vi "BalancePressure4a.vi"(0 "FirgelliError":errorcluster, 1 "length":dbl=50.0 caption="Actuator Length (mm)", 2 "DesiredPressure":dbl=-0.08 min=-1.0 max=0.0 step=0.001, 3 "Position (mm)":dbl(slide)=25.0 min=0.0 max=50.0 step=0.2 scale=0.0..50.0 scale format="%.2f", 4 "ArduinoHandle":T2={"VISA resource"="", "Board Type"=enum."Uno", "Connection Type"=enum."USB / Serial", "Bytes Per Packet (15)"=15}, 5 "CurrentPressure":dbl, 6 "WRITE_HANDLE":u32 format="%04x", 7 "PressureOffset":dbl, 8 "READ_HANDLE":u32 format="%04x", 9 "Control Values":T1, 10 "Transducer (psi)":dbl(ring)=1.0 items=["+/- .18 psi"=1.0, "+/- .36 psi"=2.0, "+/- 1.08 psi"=3.0], 11 "Syringe (mL)":dbl(ring)=1.0 items=[".5 mL"=2.0, "1 mL"=1.0, "3 mL"=3.0]) -> (14 "FirgelliError Out":errorcluster, 15 "Control Values Out":T1, 16 "UpdateChart?":bool, 17 "Position (mm) Out":dbl(slide)=25.0 min=0.0 max=50.0 step=0.2 scale=0.0..50.0 scale format="%.2f", 18 "ArduinoError Out":errorcluster, 19 "Pressure (psi)":dbl)   [LabVIEW 2011]
uses:
  <vilib>/LabVIEW Interface for Arduino/Type Defs/Arduino Resource.ctl
  <vilib>/LabVIEW Interface for Arduino/Type Defs/Board Type.ctl
  orders/Firgelli motor/LAC_Software_V2/Firgelli Labview Example/Firgelli_LAC_LabVIEWsourceVer8_2/typeDefs/controlValues.ctl
  <vilib>/LabVIEW Interface for Arduino/LabVIEW Interface for Arduino.lvlib
panel:
  in  "Accuracy":dbl
  in  "P":dbl=4.0
  in  "stop 2":bool
  in  "stop":bool
  in  "D":dbl
  in  "I":dbl
  out "LastError":dbl
  out "Error":dbl
  out "LastPressure":dbl
  in  "ArduinoError":errorcluster
  in  "Analog Input Pin (0)":u8=1
  in  "Valve I/O Pin":u8=2
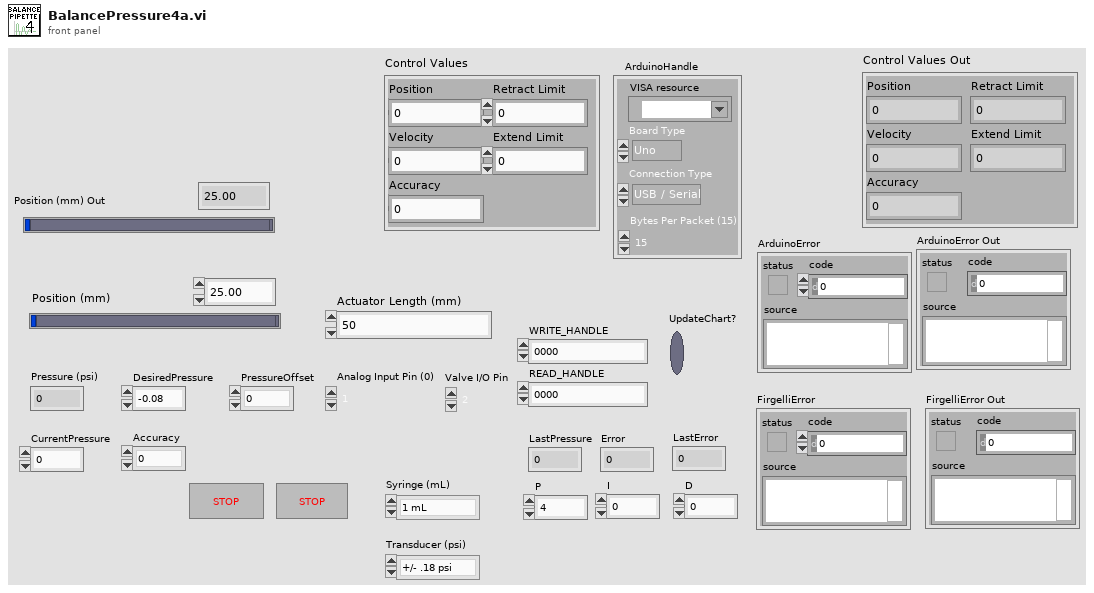
[diagram p1: front panel]
types:
  T1 = typedef "controlValues.ctl" = cluster{"Position":u16, "Velocity":u16, "Accuracy":u16, "Retract Limit":u16, "Extend Limit":u16}
  T2 = typedef "LabVIEW Interface for Arduino.lvlib/Arduino Resource.ctl" = cluster{"VISA resource":refnum<visa-resource-name>, "Board Type":T3, "Connection Type":enum8{"USB / Serial"}, "Bytes Per Packet (15)":u8}
  T3 = typedef "LabVIEW Interface for Arduino.lvlib/Board Type.ctl" = enum16{"Uno", "Dimuelanove w/Atmega 328", "Mega 2560"}
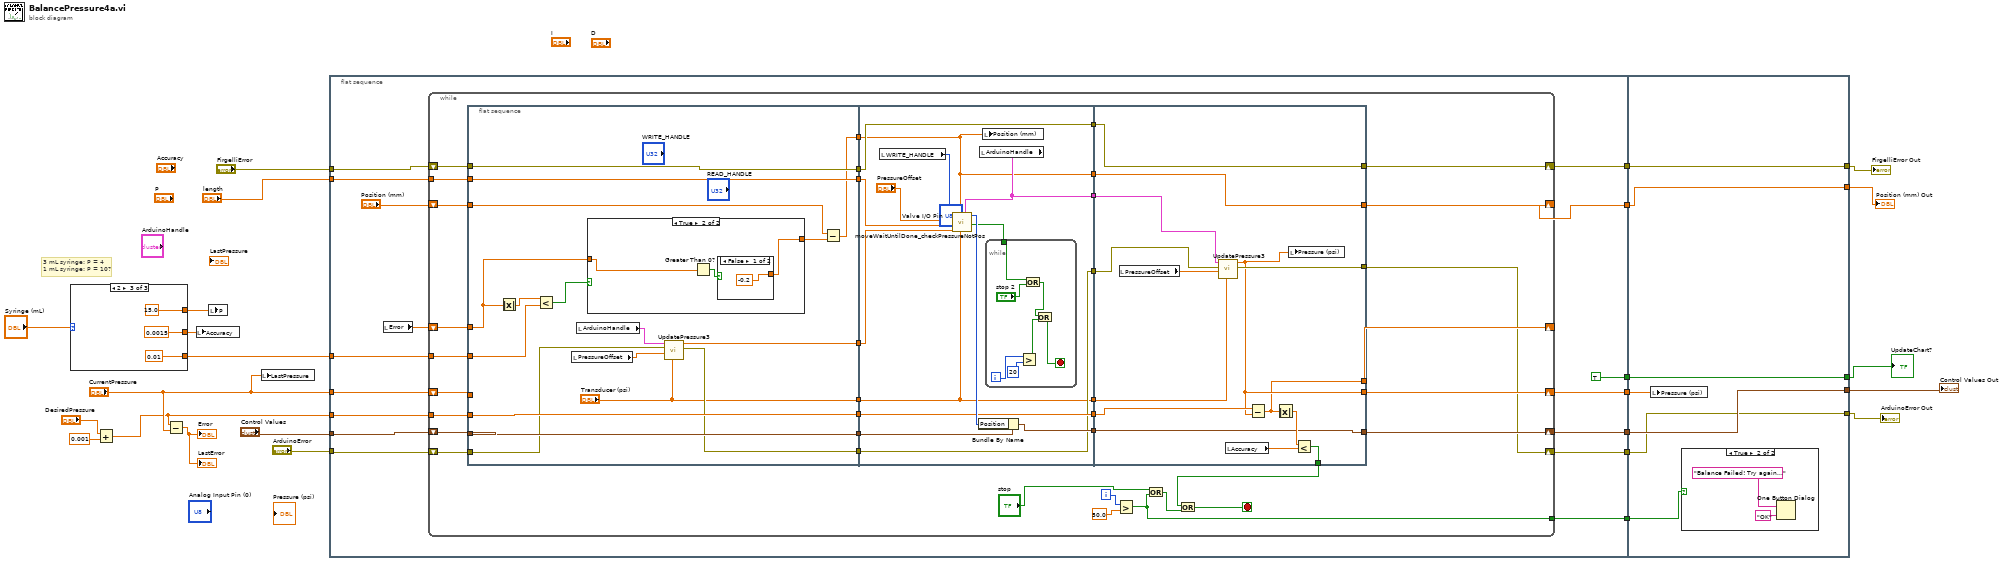
[diagram p0: block diagram]
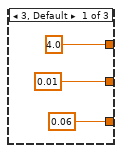
[diagram p2: hidden frame]
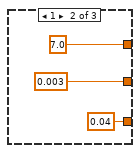
[diagram p3: hidden frame]
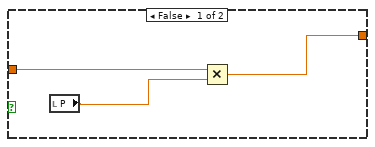
[diagram p4: hidden frame]
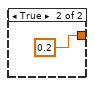
[diagram p5: hidden frame]
diagram:
  # "3 mL syringe: P = 4\n1 mL syringe: P = 10?"
  n1 = case shown="2" "Syringe (mL)" {
    tunnel: [4.0 ("P") 7.0 ("P") 15.0 ("P")] -> w6
    tunnel: [0.01 ("Accuracy") 0.003 ("Accuracy") 0.0015 ("Accuracy")] -> w5
    tunnel: [0.06 0.04 0.01] -> w4
    frame 3, Default {
    }
    frame 1 {
    }
    frame 2 {
    }
  }
  n2 = Add(x="DesiredPressure", y=0.001) -> (x+y=w1:dbl)
  n3 = Subtract(x=w1, y="CurrentPressure") -> (x-y=→"Error" →"LastError":dbl)
  n4 = local write "Accuracy"(w5) -> ()
  n5 = local write "P"(w6) -> ()
  n6 = local write "LastPressure"("CurrentPressure") -> ()
  n7 = flat-sequence {
    tunnel: "CurrentPressure" -> [w50]
    tunnel: "FirgelliError" -> [w49]
    tunnel: "Control Values" -> [w48]
    tunnel: [w47] -> w25
    tunnel: [TRUE] -> w24
    tunnel: [w45] -> w23
    tunnel: [w44] -> w22
    tunnel: [w43] -> w21
    tunnel: [w36] -> w20
    tunnel: "ArduinoError" -> [w42]
    tunnel: w1 -> [w41]
    tunnel: [w39] -> w11
    tunnel: "length" -> [w37]
    tunnel: w4 -> [w35]
    tunnel: [w151] -> w15
    tunnel: [w152] -> w14
    tunnel: [w153] -> w13
    tunnel: [w154] -> w19
    tunnel: w25 -> [w150]
    tunnel: w24 -> [w154]
    tunnel: w23 -> [w153]
    tunnel: w22 -> [w152]
    tunnel: w21 -> [w151]
    tunnel: w20 -> [w149]
    tunnel: [w149] -> w12
    tunnel: w11 -> [w148]
    frame #0 {
      n8 = local read "Error"() -> (w38:dbl)
      n9 = while {
        shift-right: [w75] -> w47
        shift-left: w50 -> [w56]
        shift-right: [w57] -> w43
        shift-left: w49 -> [w83]
        tunnel: w37 -> [w81]
        shift-right: [w78] -> w45
        shift-left: w48 -> [w79]
        shift-right: [w68] -> w44
        shift-left: w42 -> [w76]
        tunnel: w41 -> [w86]
        shift-right: [w70] -> _
        shift-left: w38 -> [w73]
        tunnel: [w67] -> w39
        shift-right: [w69] -> w36
        shift-left: "Position (mm)" -> [w87]
        tunnel: w35 -> [w51]
        i -> [w72]
        stop <- w63 stop-if-true
        n10 = flat-sequence {
          tunnel: w87 -> [w100]
          tunnel: w86 -> [w101]
          tunnel: [w95] -> w85
          tunnel: [w104] -> w84
          tunnel: w83 -> [w104]
          tunnel: [w103] -> w82
          tunnel: w81 -> [w103]
          tunnel: [w102] -> w80
          tunnel: w79 -> [w102]
          tunnel: [w91] -> w77
          tunnel: w76 -> [w92]
          tunnel: [w101] -> w74
          tunnel: w73 -> [w96]
          tunnel: w56 -> [_]
          tunnel: [w93] -> w54
          tunnel: ["Transducer (psi)"] -> w52
          tunnel: w51 -> [w88]
          tunnel: w85 -> [w114]
          tunnel: [w114] -> w62
          tunnel: w84 -> [w118]
          tunnel: w82 -> [w123]
          tunnel: w80 -> [w126]
          tunnel: [w125] -> w61
          tunnel: w77 -> [w120]
          tunnel: [w120] -> w60
          tunnel: w74 -> [w121]
          tunnel: [w121] -> w59
          tunnel: [w118] -> w58
          tunnel: [w116] -> w55
          tunnel: w54 -> [w115]
          tunnel: [w113] -> w53
          tunnel: w52 -> [w113]
          tunnel: w62 -> [w147]
          tunnel: w61 -> [w142]
          tunnel: w60 -> [w144]
          tunnel: w59 -> [w140]
          tunnel: [w141] -> w66
          tunnel: [w147] -> w69
          tunnel: [w142] -> w78
          tunnel: [w145] -> w68
          tunnel: [w139] -> w75
          tunnel: [w138] -> w70
          tunnel: w58 -> [w137]
          tunnel: [w137] -> w57
          tunnel: w55 -> [w136]
          tunnel: w53 -> [w134]
          frame #0 {
            n11 = Absolute Value(x=w96) -> (abs(x)=w99:dbl)
            n12 = Less?(x=w99, y=w88) -> (x < y?=w98:bool)
            n13 = local read "PressureOffset"() -> (w90:dbl)
            n14 = local read "ArduinoHandle"() -> (w94:T2)
            n15 = case shown="True" w98 {
              tunnel: [w107 w109] -> w97
              tunnel: w96 -> [w106 w108]
              frame False {
                n16 = local read "P"() -> (w105:dbl)
                n17 = Multiply(x=w106, y=w105) -> (x*y=w107:dbl)
              }
              frame True {
                n18 = Greater Than 0?(x=w108) -> (x > 0?=w110:bool)
                n19 = case shown="False" w110 {
                  tunnel: [-0.2 0.2] -> w109
                  frame False {
                  }
                  frame True {
                  }
                }
              }
            }
            n20 = call "UpdatePressure3.vi"("Syringe (mL)"="Transducer (psi)", "PressureOffset"=w90, "Arduino error in"=w92, "ArduinoHandle"=w94) -> ("Arduino error out"=w91:errorcluster, "Pressure (psi)"=w93:dbl)  [unwired: 6 in]
            n21 = Subtract(x=w100, y=w97) -> (x-y=w95:dbl)
          }
          frame #1 {
            n22 = local read "WRITE_HANDLE"() -> (w124:u32)
            n23 = local read "ArduinoHandle"() -> (w116:T2)
            n24 = call "moveWaitUntilDone_checkPressureNotPos.vi"("ArduinoHandle"=w116, "Analog Input Pin (0)"=w113, "Position (mm)"=w114, "Pressure (psi)"=w115, "maxLength"=w123, "PressureOffset"="PressureOffset", "WRITE_HANDLE"=w124) -> ("moveDone?"=w119:bool, "regSetting"=w122:u16)  [unwired: 3 in]
            n25 = Bundle By Name(cluster=w126, "Position"=w122) -> (w125:T1)
            n26 = local write "Position (mm)"(w114) -> ()
            n27 = while {
              tunnel: w119 -> [w133]
              i -> [w130]
              stop <- w127 stop-if-true
              n28 = Greater?(x=w130, y=20) -> (0:w128:bool)
              n29 = Or(x=w133, y="stop 2") -> (x .or. y?=w131:bool)
              n30 = Or(x=w131, y=w128) -> (x .or. y?=w127:bool)
            }
          }
          frame #2 {
            n31 = local read "PressureOffset"() -> (w143:dbl)
            n32 = call "UpdatePressure3.vi"("Syringe (mL)"=w134, "PressureOffset"=w143, "Arduino error in"=w144, "ArduinoHandle"=w136) -> ("Arduino error out"=w145:errorcluster, "Pressure (psi)"=w139:dbl)  [unwired: 6 in]
            n33 = local read "Accuracy"() -> (w135:dbl)
            n34 = Subtract(x=w140, y=w139) -> (x-y=w138:dbl)
            n35 = Absolute Value(x=w138) -> (abs(x)=w146:dbl)
            n36 = local write "Pressure (psi)"(w139) -> ()
            n37 = Less?(x=w146, y=w135) -> (x < y?=w141:bool)
          }
        }
        n38 = Greater?(x=w72, y=50.0) -> (0:w67:bool)
        n39 = Or(x="stop", y=w67) -> (x .or. y?=w64:bool)
        n40 = Or(x=w66, y=w64) -> (x .or. y?=w63:bool)
      }
    }
    frame #1 {
      n41 = local write "Pressure (psi)"(w150) -> ()
      n42 = case shown="True" w148 {
        frame False {
        }
        frame True {
          n43 = One Button Dialog(message="Balance Failed! Try again...", button name ("OK")="OK") -> ()  [unwired: 1 out]
        }
      }
    }
  }
  "UpdateChart?" <- w19
  "ArduinoError Out" <- w14
  "FirgelliError Out" <- w15
  "Control Values Out" <- w13
  "Position (mm) Out" <- w12
